vi "E06_Variables_Locales.vi"() -> ()   [LabVIEW 2026]
panel:
  in  "stop":bool
  out "Numeric 2":dbl
  out "Numeric":dbl
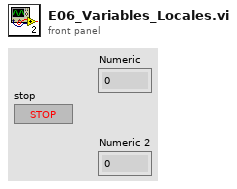
[diagram p1: front panel]
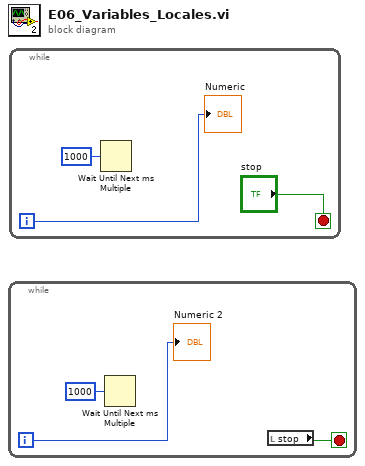
[diagram p0: block diagram]
diagram:
  n1 = while {
    i -> [w3]
    stop <- w1 stop-if-true
    n2 = Wait Until Next ms Multiple(millisecond multiple=u32 1000) -> ()  [unwired: 1 out]
    n3 = local read "stop"() -> (w1:bool)
    "Numeric 2" <- w3
  }
  n4 = while {
    i -> [w6]
    stop <- "stop" stop-if-true
    n5 = Wait Until Next ms Multiple(millisecond multiple=u32 1000) -> ()  [unwired: 1 out]
    "Numeric" <- w6
  }
